vi "PhotonTrackedTarget_PopulatePacket.vi"(11 "TrackedTarget":T1={"Yaw"=0.0, "Pitch"=0.0, "Area"=0.0, "Skew"=0.0, "TargetCorners"=[], "CameraToTarget"={"TRANSLATION"={"X"=0.0, "Y"=0.0}, "ROTATION"={"VALUE"=0.0, "COS"=1.0, "SIN"=0.0}, "xF"=FALSE}, "FiducialId"=0} {"CameraToTarget"."ROTATION"."SIN" format="%13.4f"; "CameraToTarget"."ROTATION"."COS" format="%13.4f"; "CameraToTarget"."ROTATION"."VALUE" format="%13.4f"; "CameraToTarget"."TRANSLATION"."Y" format="%14.3f"; "CameraToTarget"."TRANSLATION"."X" format="%14.3f"}) -> (3 "RawData Out":u8[](array[numeric]))   [LabVIEW 2020, in "PhotonVisionLib.lvlib"]
doc: "Encode a TrackedTarget cluster into an array of bytes.\n\nInputs:\n - TrackedTarget -- TrackedTarget cluster.\n\nOutputs:\n - RawDataOut -- Byte array containing the encoded data."
uses:
  PhotonVisionLib.lvlib
  TypeDef/PhotonTrackedTargetType.ctl
  TypeDef/TargetCornerType.ctl
  <vilib>/Rock Robotics/WPI/ThirdParty/JAS_Junk/TrajLib/TypeDef/TRANSFORM2D.ctl
  <vilib>/Rock Robotics/WPI/ThirdParty/JAS_Junk/TrajLib/TypeDef/TRANSLATION2D.ctl
  <vilib>/Rock Robotics/WPI/ThirdParty/JAS_Junk/TrajLib/TypeDef/ROTATION2D.ctl
  <vilib>/Rock Robotics/WPI/ThirdParty/JAS_Junk/TrajLib/Trajectory_Library.lvlib
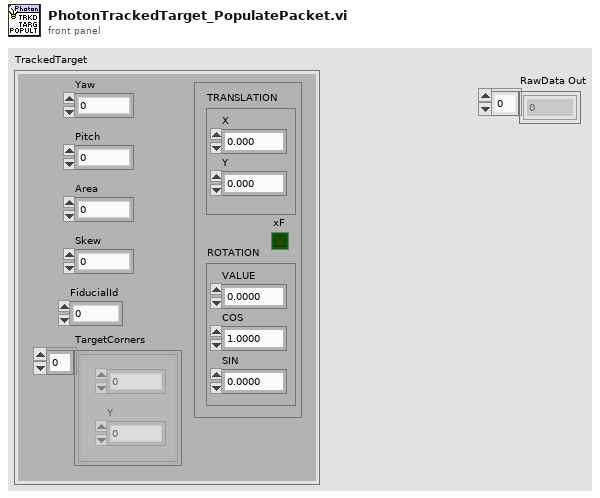
[diagram p1: front panel]
types:
  T1 = typedef "PhotonVisionLib.lvlib/PhotonTrackedTargetType.ctl" = cluster{"Yaw":dbl, "Pitch":dbl, "Area":dbl, "Skew":dbl, "TargetCorners":T2[], "CameraToTarget":T3, "FiducialId":i32}
  T2 = typedef "PhotonVisionLib.lvlib/TargetCornerType.ctl" = cluster{"X":dbl, "Y":dbl}
  T3 = typedef "Trajectory_Library.lvlib/TRANSFORM2D.ctl" = cluster{"TRANSLATION":T4, "ROTATION":T5, "xF":bool}
  T4 = typedef "Trajectory_Library.lvlib/TRANSLATION2D.ctl" = cluster{"X":dbl, "Y":dbl}
  T5 = typedef "Trajectory_Library.lvlib/ROTATION2D.ctl" = cluster{"VALUE":dbl, "COS":dbl, "SIN":dbl}
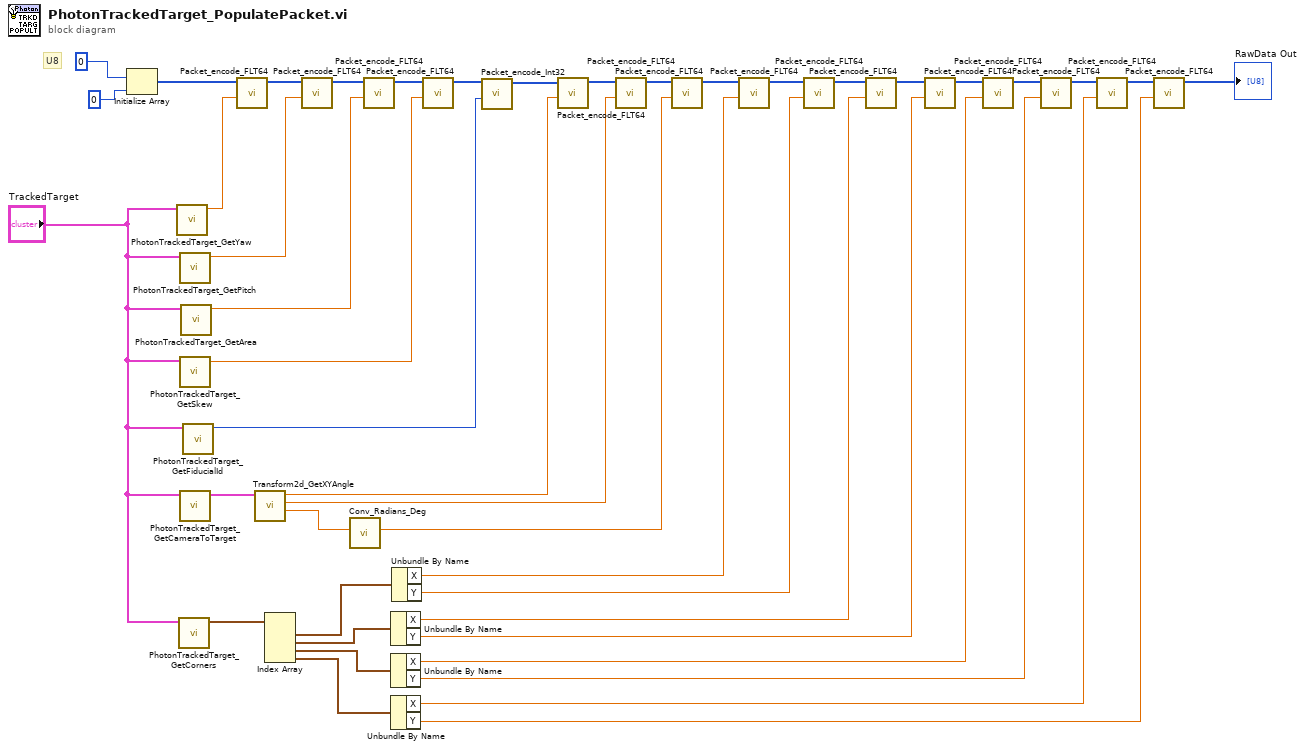
[diagram p0: block diagram]
diagram:
  # "U8"
  n1 = Initialize Array(u8 0 ("element"), 0 ("dimension size")) -> (w39:u8[])
  n2 = call "PhotonTrackedTarget_GetYaw.vi"("TrackedTarget"="TrackedTarget") -> ("Yaw"=w33:dbl)  [unwired: 10 in]
  n3 = call "PhotonTrackedTarget_GetCorners.vi"("TrackedTarget"="TrackedTarget") -> ("TargetCorners"=w26:T2[])  [unwired: 10 in]
  n4 = call "PhotonTrackedTarget_GetPitch.vi"("TrackedTarget"="TrackedTarget") -> ("Pitch"=w32:dbl)  [unwired: 10 in]
  n5 = call "PhotonTrackedTarget_GetSkew.vi"("TrackedTarget"="TrackedTarget") -> ("Skew"=w30:dbl)  [unwired: 10 in]
  n6 = call "PhotonTrackedTarget_GetCameraToTarget.vi"("TrackedTarget"="TrackedTarget") -> ("CameraToTarget"=w41:T3)  [unwired: 10 in]
  n7 = call "PhotonTrackedTarget_GetArea.vi"("TrackedTarget"="TrackedTarget") -> ("Area"=w31:dbl)  [unwired: 10 in]
  n8 = call "PhotonTrackedTarget_GetFiducialId.vi"("TrackedTarget"="TrackedTarget") -> ("FiducialId"=w1:i32)  [unwired: 10 in]
  n9 = call "Packet_encode_FLT64.vi"("FLT64_Value"=w33, "RawData In"=w39) -> ("RawData Out"=w38:u8[])  [unwired: 9 in]
  n10 = call <vilib>:"Transform2d_GetXYAngle.vi"("inTRANSFORM"=w41) -> ("Angle"=w40:dbl, "Y"=w28:dbl, "X"=w29:dbl)  [unwired: 8 in]
  n11 = Index Array(array=w26) -> (element #1=w25:T2, element #2=w24:T2, element #3=w23:T2, element #4=w22:T2)  [unwired: 4 in]
  n12 = call "Packet_encode_FLT64.vi"("FLT64_Value"=w32, "RawData In"=w38) -> ("RawData Out"=w37:u8[])  [unwired: 9 in]
  n13 = call <vilib>:"Conv_Radians_Deg.vi"("Radians"=w40) -> ("Degrees"=w27:dbl)  [unwired: 10 in]
  n14 = call "Packet_encode_FLT64.vi"("FLT64_Value"=w31, "RawData In"=w37) -> ("RawData Out"=w36:u8[])  [unwired: 9 in]
  n15 = Unbundle By Name(w24) -> ("X"=w11:dbl, "Y"=w10:dbl)
  n16 = Unbundle By Name(w23) -> ("X"=w9:dbl, "Y"=w8:dbl)
  n17 = Unbundle By Name(w22) -> ("X"=w7:dbl, "Y"=w6:dbl)
  n18 = Unbundle By Name(w25) -> ("X"=w13:dbl, "Y"=w12:dbl)
  n19 = call "Packet_encode_FLT64.vi"("FLT64_Value"=w30, "RawData In"=w36) -> ("RawData Out"=w3:u8[])  [unwired: 9 in]
  n20 = call "Packet_encode_Int32.vi"("Int32_Value"=w1, "RawData In"=w3) -> ("RawData Out"=w2:u8[])  [unwired: 9 in]
  n21 = call "Packet_encode_FLT64.vi"("FLT64_Value"=w29, "RawData In"=w2) -> ("RawData Out"=w35:u8[])  [unwired: 9 in]
  n22 = call "Packet_encode_FLT64.vi"("FLT64_Value"=w28, "RawData In"=w35) -> ("RawData Out"=w34:u8[])  [unwired: 9 in]
  n23 = call "Packet_encode_FLT64.vi"("FLT64_Value"=w27, "RawData In"=w34) -> ("RawData Out"=w15:u8[])  [unwired: 9 in]
  n24 = call "Packet_encode_FLT64.vi"("FLT64_Value"=w13, "RawData In"=w15) -> ("RawData Out"=w21:u8[])  [unwired: 9 in]
  n25 = call "Packet_encode_FLT64.vi"("FLT64_Value"=w12, "RawData In"=w21) -> ("RawData Out"=w20:u8[])  [unwired: 9 in]
  n26 = call "Packet_encode_FLT64.vi"("FLT64_Value"=w11, "RawData In"=w20) -> ("RawData Out"=w19:u8[])  [unwired: 9 in]
  n27 = call "Packet_encode_FLT64.vi"("FLT64_Value"=w10, "RawData In"=w19) -> ("RawData Out"=w18:u8[])  [unwired: 9 in]
  n28 = call "Packet_encode_FLT64.vi"("FLT64_Value"=w9, "RawData In"=w18) -> ("RawData Out"=w17:u8[])  [unwired: 9 in]
  n29 = call "Packet_encode_FLT64.vi"("FLT64_Value"=w8, "RawData In"=w17) -> ("RawData Out"=w16:u8[])  [unwired: 9 in]
  n30 = call "Packet_encode_FLT64.vi"("FLT64_Value"=w7, "RawData In"=w16) -> ("RawData Out"=w14:u8[])  [unwired: 9 in]
  n31 = call "Packet_encode_FLT64.vi"("FLT64_Value"=w6, "RawData In"=w14) -> ("RawData Out"=→"RawData Out":u8[])  [unwired: 9 in]
